vi "Sequence Delete.vi"(8 "error in (no error)":errorcluster, 10 "Sequence ID":string, 11 "Connection Refnum":T1) -> (0 "error out":errorcluster, 3 "Connection Refnum":T1)   [LabVIEW 2011]
uses:
  SI.LIB/ODBC/SQL Controls/Connection Refnum.ctl
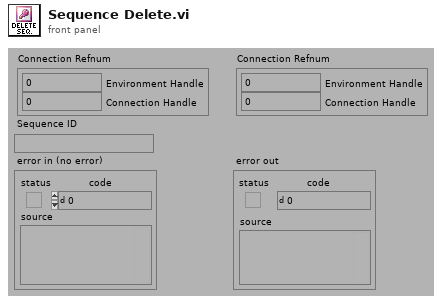
[diagram p1: front panel]
types:
  T1 = typedef "Connection Refnum.ctl" = cluster{"Environment Handle":i32, "Connection Handle":i32}
  T2 = typedef "Statement Refnum.ctl" = cluster{"Statement Handle":i32, "Parameter Number":u16}
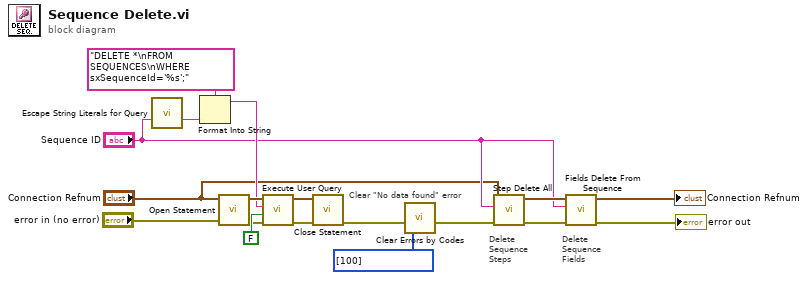
[diagram p0: block diagram]
diagram:
  # "Clear \"No data found\" error"
  # "Delete\nSequence\nFields"
  # "Delete\nSequence\nSteps"
  n1 = call "Escape String Literals for Query.vi"("String"="Sequence ID") -> ("escaped String"=w5:string)  [unwired: 1 in, 13 out]
  n2 = Format Into String(format string="DELETE *\nFROM SEQUENCES\nWHERE sxSequenceId='%s';" ("User Query"), w5) -> (resulting string=w12:string)  [unwired: 2 in, 1 out]
  n3 = call "Open Statement.vi"("error in (no error)"="error in (no error)", "Connection Refnum"="Connection Refnum") -> ("error out"=w14:errorcluster, "Statement Refnum"=w13:T2)  [unwired: 4 out]
  n4 = call "Execute User Query.vi"("error in (no error)"=w14, "Return Data? (f)"=FALSE, "User Query"=w12, "Statement Refnum"=w13) -> ("error out"=w16:errorcluster, "Statement Refnum"=w17:T2)  [unwired: 2 out]
  n5 = call "Close Statement.vi"("error in (no error)"=w16, "Statement Refnum"=w17) -> ("error out"=w8:errorcluster)  [unwired: 5 out]
  n6 = call "Clear Errors by Codes.vi"("Error Codes\nto Clear (Empty)"=i32[] [100] ("Error Codes\nto Clear (Empty)"), "error in (no error)"=w8) -> ("error out"=w7:errorcluster)  [unwired: 5 out]
  n7 = call "Step Delete All.vi"("error in (no error)"=w7, "sxSequenceId (\"\")"="Sequence ID", "Connection Refnum"="Connection Refnum") -> ("error out"=w10:errorcluster, "Connection Refnum"=w11:T1)  [unwired: 7 out]
  n8 = call "Fields Delete From Sequence.vi"("error in (no error)"=w10, "sxSequenceId (\"\")"="Sequence ID", "Connection Refnum"=w11) -> ("error out"=→"error out":errorcluster, "Connection Refnum"=→"Connection Refnum":T1)  [unwired: 7 out]
